vi "Custom_Config_Volt_Slew.vi"(7 "Enable Voltage Slew Rate Override (False)":bool, 8 "error in (no error)":errorcluster {"code" format="%.0x"}, 9 "Voltage Slew Rate (9.9E+37 A/s)":dbl=9.9e+37 format="%^.3e", 10 "Channel Name (1)":string="1", 11 "VISA resource name":refnum<visa-resource-name>) -> (0 "error out":errorcluster {"code" format="%.0x"}, 3 "VISA resource name out":refnum<visa-resource-name>)   [LabVIEW 2019, in "6700C.lvlib" / "6700C.lvclass"]
uses:
  Library/6700C.lvclass
  <instrlib>/Agilent N6700 Series/Agilent N6700 Series.lvlib
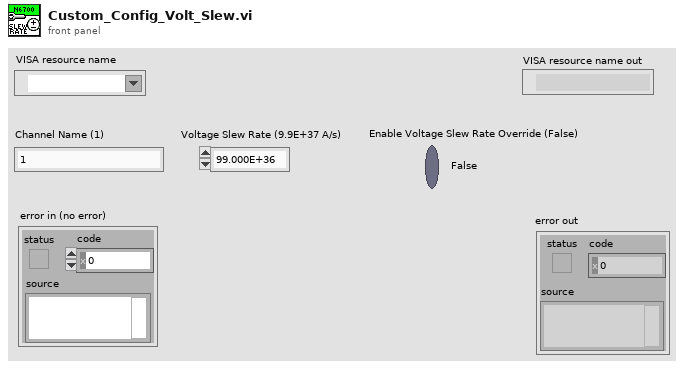
[diagram p1: front panel]
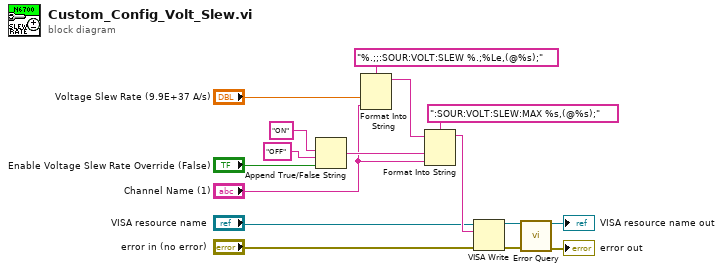
[diagram p0: block diagram]
diagram:
  n1 = Append True/False String(1:"Enable Voltage Slew Rate Override (False)", 2:"OFF", 3:"ON") -> (0:w14:string)  [unwired: 1 in]
  n2 = Format Into String(format string="%.;;:SOUR:VOLT:SLEW %.;%Le,(@%s);", "Voltage Slew Rate (9.9E+37 A/s)", "Channel Name (1)") -> (resulting string=w11:string)  [unwired: 2 in, 1 out]
  n3 = Format Into String(format string=":SOUR:VOLT:SLEW:MAX %s,(@%s);", initial string=w11, w14, "Channel Name (1)") -> (resulting string=w8:string)  [unwired: 1 in, 1 out]
  n4 = VISA Write(VISA resource name="VISA resource name", write buffer=w8, error in (no error)="error in (no error)") -> (VISA resource name out=w5:refnum<visa-resource-name>, error out=w6:errorcluster)  [unwired: 1 out]
  n5 = call <instrlib>:"Error Query.vi"("VISA resource name"=w5, "error in (no error)"=w6) -> ("VISA resource name out"=→"VISA resource name out":refnum<visa-resource-name>, "error out"=→"error out":errorcluster)  [unwired: 10 in, 2 out]
